vi "Units_DegreesToRotations.vi"(10 "Degrees":dbl) -> (2 "Rotations":dbl)   [LabVIEW 2019, in "Trajectory_Library.lvlib"]
doc: "Convert a value from degrees to rotations\n\nInputs: \n - Degrees - Angle (Degrees)\n\nOutputs:\n - Rotations - Angle (Rotations)"
uses:
  Trajectory_Library.lvlib
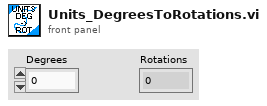
[diagram p1: front panel]
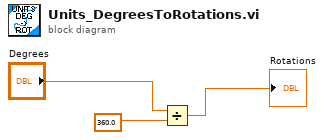
[diagram p0: block diagram]
diagram:
  n1 = Divide(x="Degrees", y=360.0) -> (x/y=→"Rotations":dbl)
